vi "Plug_In_Move_Trav_and_Meas.vi"() -> (5 "Plug in titles":string[](array[string]), 7 "Plug in values":string[](array[string]))   [LabVIEW 2018]
uses:
  Controls/Post_Process.ctl
  Gen Trav/Trav_mode.ctl
  Controls/User_Specific_mode.ctl
  Controls/Tunnel_Coordinates.ctl
  Globals/Meas_global.vi
  Globals/Trav_pos_global.vi
panel:
  in  "milliseconds to wait":u32=2500
  out "Case Currently On":string
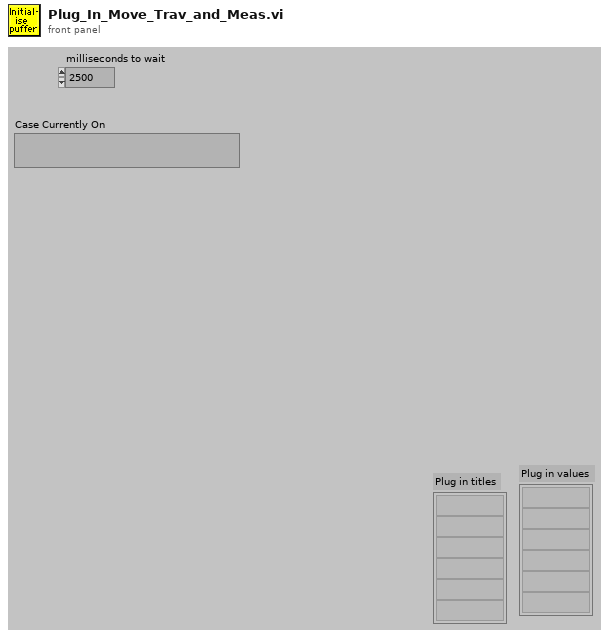
[diagram p1: front panel]
types:
  T1 = typedef "Traverse_cluster.ctl" = cluster{"Start X":sgl, "Start Y":sgl, "Start Z":sgl, "End X":sgl, "End Y":sgl, "End Z":sgl, "No. of pts.":i32, "Spacing":T2, "Filename":path, "Tunnel Speed":dbl, "Averaging time (min)":dbl, "Extra Commands":string, "Carrier_1 Q (l/min)":dbl, "Carrier_2 Q (l/min)":dbl, "Trace Gas Concentration (%)":dbl, "Specific Arguments":string, "Comments":string, "Row No":i32, "Row Type Selector":T3, "Completion time":string, "Row Duration (mins)":dbl, "No. of Valid pts.":i32, "Meas Setup File":string}
  T2 = typedef "Spacing.ctl" = enum16{"Linear", "Log", "Gauss", "Specified", "N/A"}
  T3 = typedef "Multi_run_mode.ctl" = enum16{"Move Traverse Only", "Set Tunnel Speed Only", "Set Source Only", "Set Measurement Conditions", "Single Measurement", "Vertical Profile", "Lateral Profile", "Longitudinal Profile", "Multi-Axis Profile", "Explore Volume", "Auto Calibrate", "Meas Fast FID Bkgnd", "Check Beam Power", "Scanning Valve Measurement", "Run VI Named:", "Set ADAM Ch", "Wait (minutes)", "Send Message", "Synchronize With:", "Fall Back to this Row", "Turn Off Row Repeating", "Traverse 3D Volume", "Blank Row", "Jump to Fall Back Row"}
  T4 = typedef "Post_Process.ctl" = enum16{"Take New Data", "Post Process Raw Data File"}
  T5 = typedef "Tunnel_Coordinates.ctl" = enum16{"Work in Tunnel Coordinates", "Work in Model Coordinates"}
  T6 = typedef "User_Specific_mode.ctl" = enum16{"Check VI only", "Run VI"}
  T7 = typedef "Trav_mode.ctl" = enum16{"Move traverse", "Read traverse position", "Teach Position"}
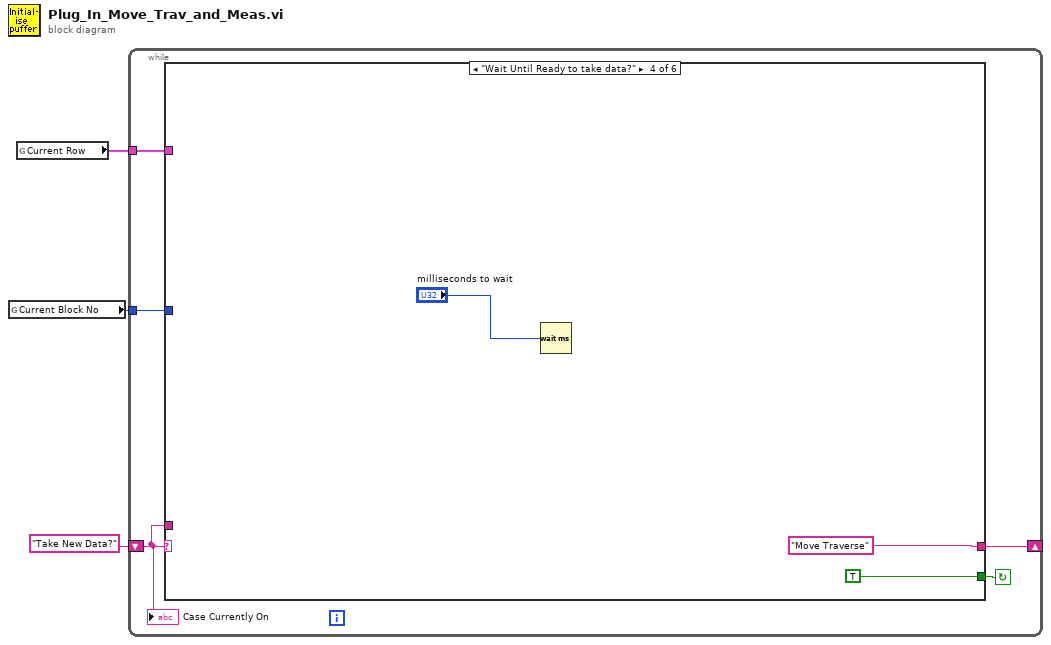
[diagram p0: block diagram]
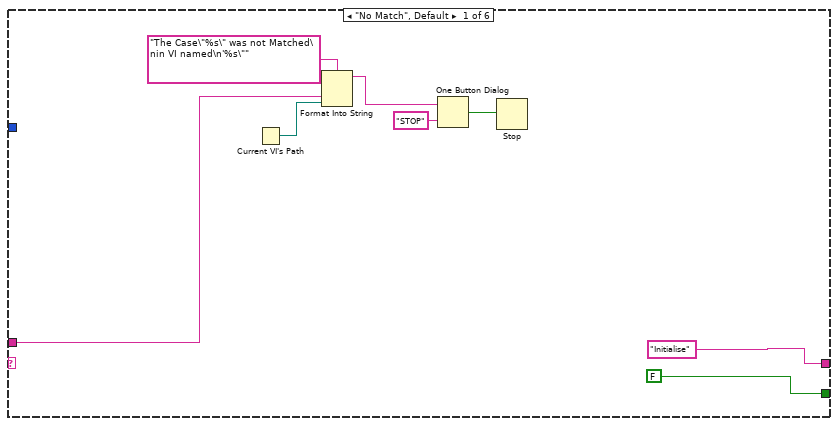
[diagram p2: hidden frame]
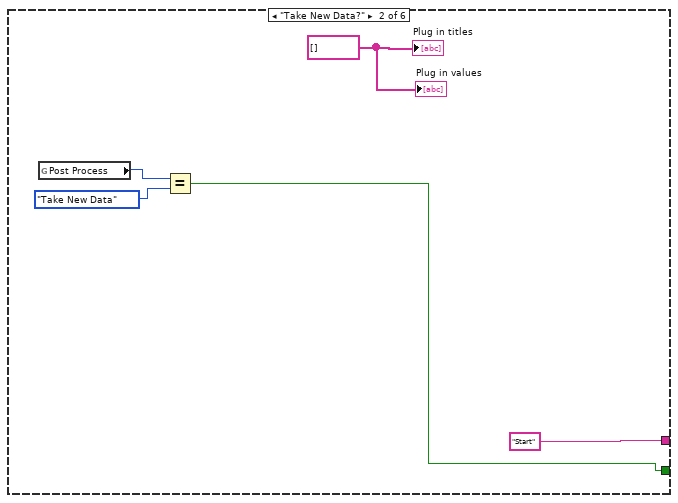
[diagram p3: hidden frame]
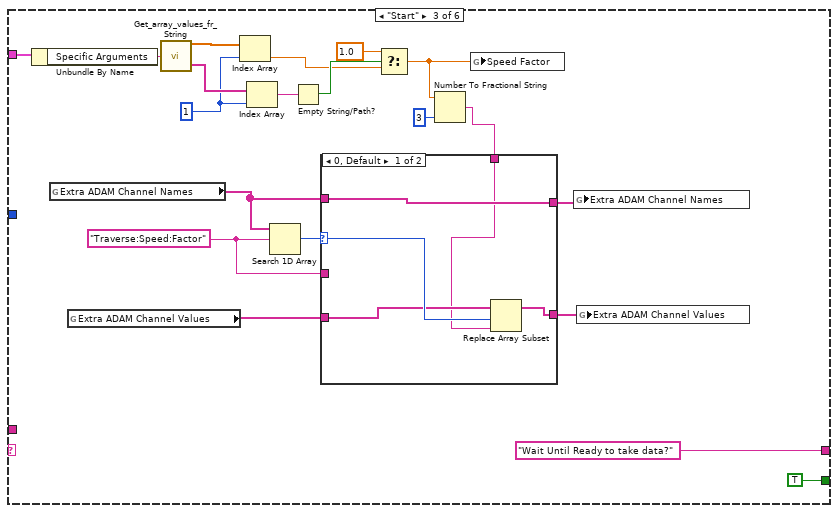
[diagram p4: hidden frame]
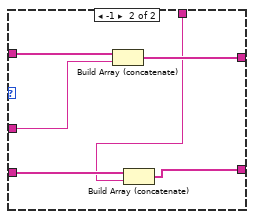
[diagram p5: hidden frame]
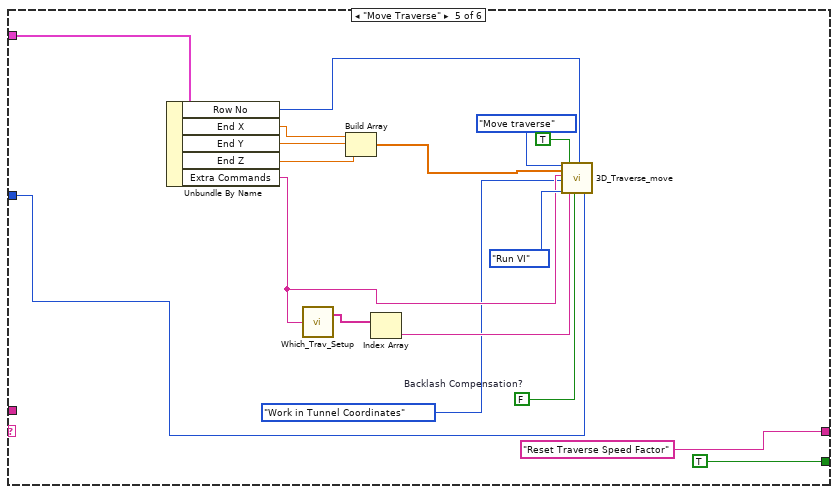
[diagram p6: hidden frame]
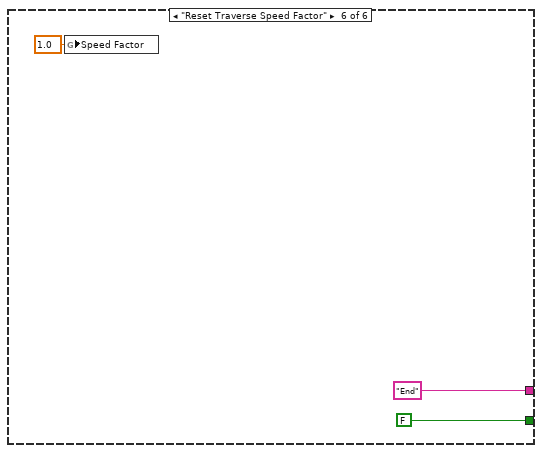
[diagram p7: hidden frame]
diagram:
  n1 = global read "Meas_global.vi" "Current Block No"() -> (w2:i32)
  n2 = global read "Trav_pos_global.vi" "Current Row"() -> (w1:T1)
  n3 = while {
    shift-left: "Take New Data?" -> [w6]
    shift-right: [w7] -> _
    tunnel: w2 -> [w5]
    tunnel: w1 -> [w4]
    stop <- w8 continue-if-true
    n4 = case shown="\"Wait Until Ready to take data?\"" w6 {
      tunnel: [FALSE w17 TRUE ("Command Found") TRUE ("Command Found") TRUE ("Command Found") FALSE ("Command Found")] -> w8
      tunnel: ["Initialise" "Start" "Wait Until Ready to take data?" ("f") "Move Traverse" "Reset Traverse Speed Factor" "End" ("f")] -> w7
      tunnel: w6 -> [w11 _ _ _ _ _]
      tunnel: w5 -> [_ _ _ _ w63 _]
      tunnel: w4 -> [_ _ w39 _ w61 _]
      frame "No Match", Default {
        n5 = Current VI's Path() -> (path=w10:path)
        n6 = Format Into String(format string="The Case\"%s\" was not Matched\nin VI named\n'%s\"" ("Format String"), w11, w10) -> (resulting string=w14:string)  [unwired: 2 in, 1 out]
        n7 = One Button Dialog(message=w14, button name ("OK")="STOP") -> (true=w12:bool)
        n8 = Stop(stop? (T)=w12) -> ()
      }
      frame "Take New Data?" {
        w18 = string[] [] ("Plug in titles")
        n9 = global read "Meas_global.vi" "Post Process"() -> (w20:T4)
        n10 = Equal?(x=w20, y=Post_Process."Take New Data" ("Post Process")) -> (x = y?=w17:bool)
        "Plug in titles" <- w18
        "Plug in values" <- w18
      }
      frame "Start" {
        w28 = "Traverse:Speed:Factor"
        w32 = 1 ("index")
        n11 = Unbundle By Name(w39) -> ("Specific Arguments"=w41:string)
        n12 = global read "Meas_global.vi" "Extra ADAM Channel Names"() -> (w29:string[])
        n13 = global read "Meas_global.vi" "Extra ADAM Channel Values"() -> (w26:string[])
        n14 = call "Get_array_values_fr_String.vi"("String Value"=w41) -> ("Numeric Array"=w40:dbl[], "String array"=w38:string[])
        n15 = Index Array(array=w40, index=w32) -> (element=w35:dbl)
        n16 = Index Array(array=w38, index=w32) -> (element=w37:string)
        n17 = Search 1D Array(1D array=w29, element=w28) -> (index of element=w30:i32)  [unwired: 1 in]
        n18 = Empty String/Path?(string/path=w37) -> (empty?=w36:bool)
        n19 = Select(t=1.0, s=w36, f=w35) -> (s? t:f=w24:dbl)
        n20 = Number To Fractional String(number=w24, precision (6)=i16 3) -> (F-format string=w22:string)  [unwired: 2 in]
        n21 = case shown="0, Default" w30 {
          selector: w30 -> [w45 _]
          tunnel: w29 -> [w46 w52]
          tunnel: w28 -> [_ w51]
          tunnel: [w46 w50] -> w27
          tunnel: w26 -> [w44 w49]
          tunnel: [w43 w48] -> w25
          tunnel: w22 -> [w42 w47]
          frame 0, Default {
            n22 = Replace Array Subset(array=w44, new element=w42, index=w45) -> (w43:string[])
          }
          frame -1 {
            n23 = Build Array (concatenate)(w52, w51) -> (w50:string[])
            n24 = Build Array (concatenate)(w49, w47) -> (w48:string[])
          }
        }
        n25 = global write "Trav_pos_global.vi" "Speed Factor"(w24) -> ()
        n26 = global write "Meas_global.vi" "Extra ADAM Channel Names"(w27) -> ()
        n27 = global write "Meas_global.vi" "Extra ADAM Channel Values"(w25) -> ()
      }
      frame "Wait Until Ready to take data?" {
        n28 = Wait (ms)(milliseconds to wait="milliseconds to wait") -> ()  [unwired: 1 out]
      }
      frame "Move Traverse" {
        w70 = FALSE  # Backlash Compensation?
        n29 = Unbundle By Name(w61) -> ("Row No"=w62:i32, "End X"=w68:sgl, "End Y"=w67:sgl, "End Z"=w66:sgl, "Extra Commands"=w58:string)
        n30 = call "Which_Trav_Setup.vi"("Extra Command String"=w58) -> ("Traverse Setups"=w60:string[])  [unwired: 2 out]
        n31 = Build Array(w68, w67, w66) -> (w69:sgl[])
        n32 = Index Array(array=w60) -> (element=w59:string)  [unwired: 1 in]
        n33 = call "3D_Traverse_move.vi"("Mode"=Trav_mode."Move traverse", "Position"=w69, "Extra command String"=w58, "Work in Tunnel Coordinates"=Tunnel_Coordinates."Work in Tunnel Coordinates", "Simulate/Run"=User_Specific_mode."Run VI", "Route Checking?"=TRUE, "Traverse name"=w59, "Backlash Compensation?"=w70, "Row Number"=w62, "Currently on Point"=w63) -> ()  [unwired: 6 in, 4 out]
      }
      frame "Reset Traverse Speed Factor" {
        n34 = global write "Trav_pos_global.vi" "Speed Factor"(1.0 ("Speed Factor")) -> ()
      }
    }
    "Case Currently On" <- w6
  }
